vi "Solve Linear Equations (EXT).vi"(6 "Tolerance":dbl=0.001 format="%#_13g", 10 "b":ext[](array[numeric]), 11 "A":ext[][](array[numeric])) -> (3 "X":ext[](array[numeric]))   [LabVIEW 2023, in "d24.lvlib"]
uses:
  d24.lvlib
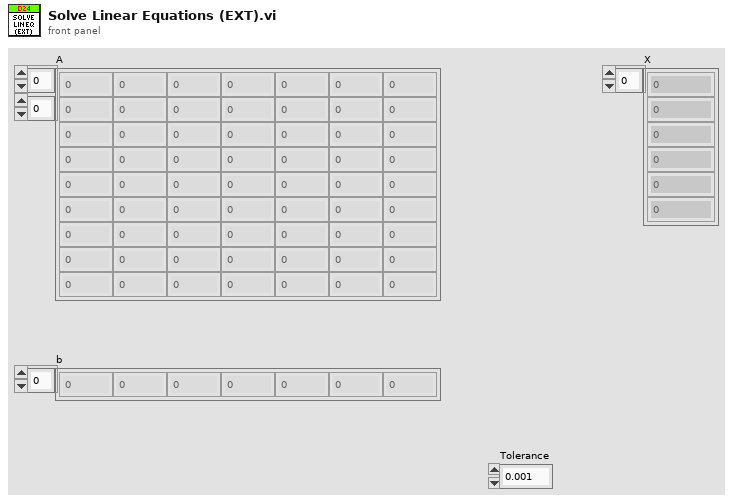
[diagram p1: front panel]
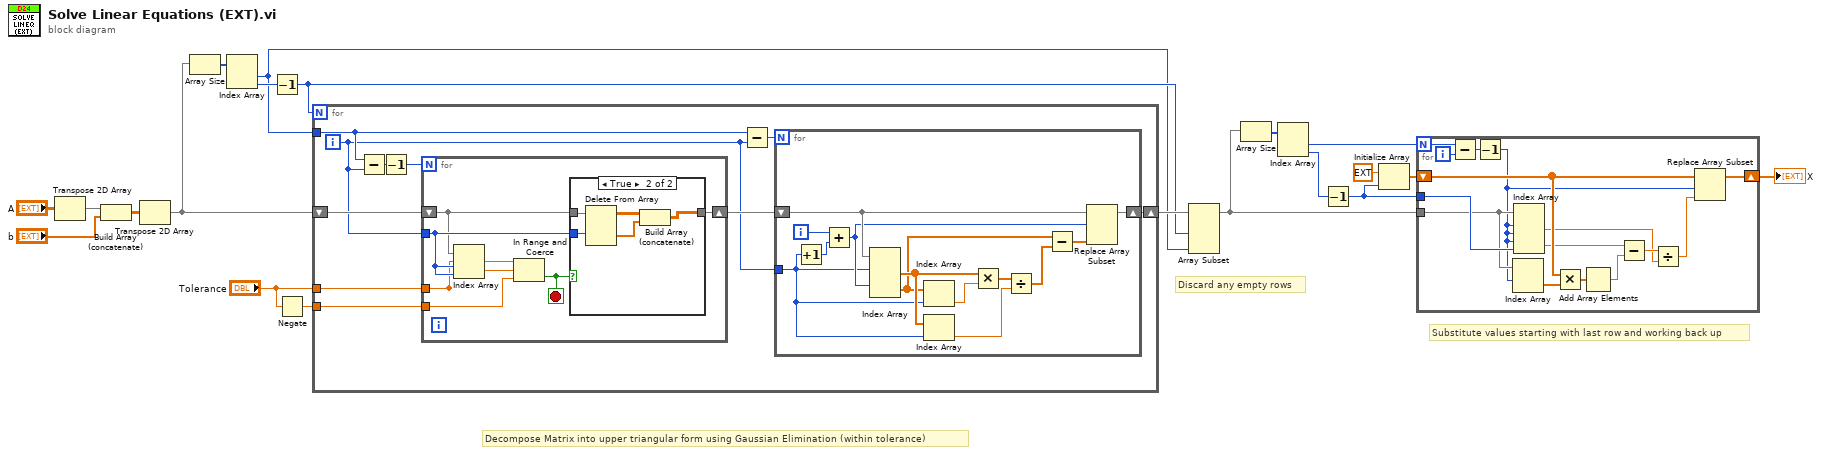
[diagram p0: block diagram]
diagram:
  # "Discard any empty rows"
  # "Substitute values starting with last row and working back up"
  # "Decompose Matrix into upper triangular form using Gaussian Elimination (within tolerance)"
  n1 = Transpose 2D Array(2D array="A") -> (transposed array=w5:ext[][])
  n2 = Build Array (concatenate)(w5, "b") -> (w4:ext[][])
  n3 = Transpose 2D Array(2D array=w4) -> (transposed array=w3:ext[][])
  n4 = Array Size(array=w3) -> (size(s)=w20:i32[])
  n5 = Index Array(array=w20) -> (element #1=w9:i32, element #2=w19:i32)  [unwired: 2 in]
  n6 = Decrement(x=w19) -> (x-1=w10:i32)
  n7 = Negate(x="Tolerance") -> (-x=w2:dbl)
  n8 = for {
    N: w10 -> [_]
    tunnel: w9 -> [w23]
    shift-right: [w30] -> w18
    shift-left: w3 -> [w28]
    tunnel: "Tolerance" -> [w26]
    tunnel: w2 -> [w25]
    i -> [w22]
    n9 = Subtract(x=w23, y=w22) -> (x-y=w24:i32)
    n10 = Decrement(x=w24) -> (x-1=w21:i32)
    n11 = for {
      N: w21 -> [_]
      tunnel: w22 -> [w37]
      shift-right: [w35] -> w27
      shift-left: w28 -> [w36]
      tunnel: w26 -> [w33]
      tunnel: [w33] -> _
      tunnel: w25 -> [w32]
      stop <- w31 stop-if-true
      n12 = Index Array(array=w36, index (row)=w37, index (col)=w37) -> (element=w34:ext)
      n13 = In Range and Coerce(upper limit=w33, x=w34, lower limit=w32) -> (In Range?=w31:bool)  [unwired: 1 out]
      n14 = case shown="True" w31 {
        tunnel: w37 -> [_ w42]
        tunnel: w36 -> [w38 w43]
        tunnel: [w38 w39] -> w35
        frame False {
        }
        frame True {
          n15 = Delete From Array(array=w43, index (row)=w42) -> (deleted portion=w40:ext[], array with subset deleted=w41:ext[][])  [unwired: 2 in]
          n16 = Build Array (concatenate)(w41, w40) -> (w39:ext[][])
        }
      }
    }
    n17 = Subtract(x=w23, y=w22) -> (x-y=w29:i32)
    n18 = for {
      N: w29 -> [_]
      tunnel: w22 -> [w47]
      shift-right: [w52] -> w30
      shift-left: w27 -> [w53]
      i -> [w49]
      n19 = Increment(x=w47) -> (x+1=w48:i32)
      n20 = Add(x=w49, y=w48) -> (x+y=w50:i32)
      n21 = Index Array(array=w53, index (row) #1=w47, index (row) #2=w50) -> (element #1=w55:ext[], element #2=w54:ext[])  [unwired: 2 in]
      n22 = Index Array(array=w54, index=w47) -> (element=w46:ext)
      n23 = Index Array(array=w55, index=w47) -> (element=w56:ext)
      n24 = Multiply(x=w55, y=w46) -> (x*y=w45:ext[])
      n25 = Divide(x=w45, y=w56) -> (x/y=w44:ext[])
      n26 = Subtract(x=w54, y=w44) -> (x-y=w51:ext[])
      n27 = Replace Array Subset(array=w53, new element=w51, index (row)=w50) -> (w52:ext[][])  [unwired: 1 in]
    }
  }
  n28 = Array Subset(array=w18, length (row)=w10, length (col)=w9) -> (w11:ext[][])  [unwired: 2 in]
  n29 = Array Size(array=w11) -> (size(s)=w17:i32[])
  n30 = Index Array(array=w17) -> (element #1=w16:i32, element #2=w8:i32)  [unwired: 2 in]
  n31 = Decrement(x=w8) -> (x-1=w7:i32)
  n32 = Initialize Array(ext 0.0, w7) -> (w13:ext[])
  n33 = for {
    N: w16 -> [w71]
    tunnel: w11 -> [w65]
    tunnel: w7 -> [w69]
    shift-right: [w68] -> w15
    shift-left: w13 -> [w67]
    i -> [w70]
    n34 = Subtract(x=w71, y=w70) -> (x-y=w62:i32)
    n35 = Decrement(x=w62) -> (x-1=w61:i32)
    n36 = Index Array(array=w65, index (row)=w61) -> (element=w64:ext[])  [unwired: 1 in]
    n37 = Index Array(array=w65, index (row) #1=w61, index (col) #1=w61, index (row) #2=w61, index (col) #2=w69) -> (element #1=w57:ext, element #2=w59:ext)
    n38 = Multiply(x=w67, y=w64) -> (x*y=w66:ext[])
    n39 = Add Array Elements(numeric array=w66) -> (sum=w58:ext)
    n40 = Subtract(x=w59, y=w58) -> (x-y=w60:ext)
    n41 = Divide(x=w60, y=w57) -> (x/y=w63:ext)
    n42 = Replace Array Subset(array=w67, new element=w63, index=w61) -> (w68:ext[])
  }
  "X" <- w15
